vi "TagConverter.vi"(11 "CVT Tags":T5[](array[typedef])) -> (3 "CVT Load Data":T1)   [LabVIEW 2020, in "Current Value Table(Rebuild).lvlib"]
uses:
  _SubVIs/TypeDefs/cvt_Tag Configuration.ctl
  _SubVIs/TypeDefs/cvt_Data Types.ctl
  Type Defs/File Format.ctl
  Type Defs/Single Tag.ctl
  Type Defs/Data Types.ctl
  Type Defs/Tag Grouping set.ctl
  Current Value Table(Rebuild).lvlib
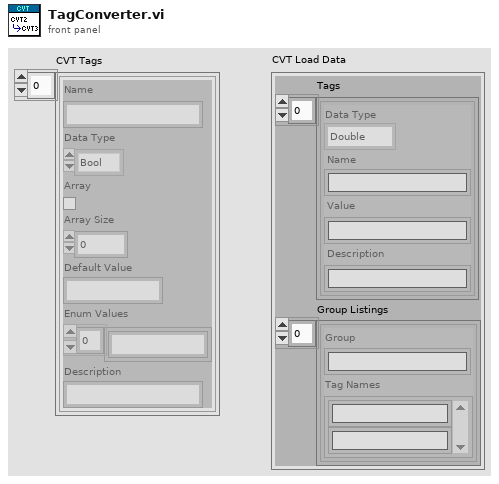
[diagram p1: front panel]
types:
  T1 = typedef "Current Value Table(Rebuild).lvlib/File Format.ctl" = cluster{"Tags":T2[], "Group Listings":T4[]}
  T2 = typedef "Current Value Table(Rebuild).lvlib/Single Tag.ctl" = cluster{"Data Type":T3, "Name":string, "Value":string, "Description":string}
  T3 = typedef "Current Value Table(Rebuild).lvlib/Data Types.ctl" = enum16{"Double", "Single", "I64", "I32", "I16", "I8", "U64", "U32", "U16", "U8", "String", "Boolean", "Array of U8", "Array of U16", "Array of U32", "Array of U64", "Array of I64", "Array of I32", "Array of I16", "Array of I8", "Array of Double", "Array of Single", "Array of Boolean", "Array of String"}
  T4 = typedef "Current Value Table(Rebuild).lvlib/Tag Grouping set.ctl" = cluster{"Group":string, "Tag Names":string[]}
  T5 = typedef "Current Value Table(Rebuild).lvlib/cvt_Tag Configuration.ctl" = cluster{"Name":string, "Data Type":T6, "Array":bool, "Size":u32, "Default":string, "Enum":string[], "Description":string}
  T6 = typedef "Current Value Table(Rebuild).lvlib/cvt_Data Types.ctl" = enum16{"Bool", "U8", "I32", "Double", "String", "Enum"}
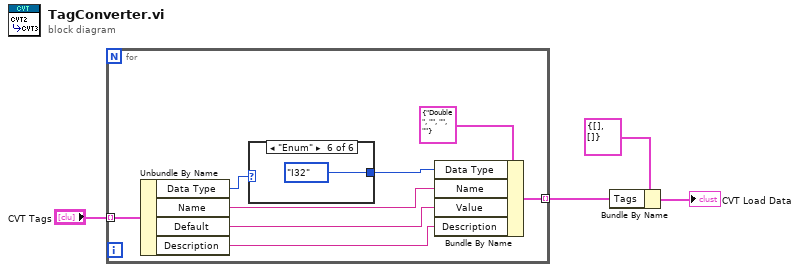
[diagram p0: block diagram]
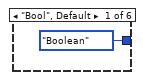
[diagram p2: hidden frame]
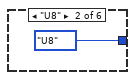
[diagram p3: hidden frame]
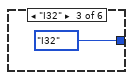
[diagram p4: hidden frame]
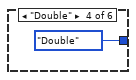
[diagram p5: hidden frame]
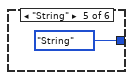
[diagram p6: hidden frame]
diagram:
  n1 = for {
    tunnel: "CVT Tags" -> [w12] mode=indexing
    tunnel: [w6] -> w1 mode=indexing
    n2 = Unbundle By Name(w12) -> ("Data Type"=w7:T6, "Name"=w10:string, "Default"=w11:string, "Description"=w9:string)
    n3 = case shown="\"Enum\"" w7 {
      tunnel: [Data_Types."Boolean" ("Data Type") Data_Types."U8" ("Data Type") Data_Types."I32" ("Data Type") Data_Types."Double" ("Data Type") Data_Types."String" ("Data Type") Data_Types."I32" ("Data Type")] -> w5
      frame "Bool", Default {
      }
      frame "U8" {
      }
      frame "I32" {
      }
      frame "Double" {
      }
      frame "String" {
      }
      frame "Enum" {
      }
    }
    n4 = Bundle By Name(cluster=T2 {"Data Type"=enum."Double", "Name"="", "Value"="", "Description"=""} ("Tag"), "Data Type"=w5, "Name"=w10, "Value"=w11, "Description"=w9) -> (w6:T2)
  }
  n5 = Bundle By Name(cluster=T1 {"Tags"=[], "Group Listings"=[]} ("CVT File Data"), "Tags"=w1) -> (→"CVT Load Data":T1)
